vi "Furnace PID Furnance only 20150313.vi"(6 "PID gains":T1={"proportional gain (Kc)"=1.0, "integral time (Ti, min)"=0.1, "derivative time (Td, min)"=0.0}, 9 "PV Furnace degC":dbl format="%.2f", 11 "SP Furnace DegC":dbl format="%.2f") -> (2 "Furnace SP":dbl format="%.2f")   [LabVIEW 2014]
uses:
  <vilib>/addons/control/pid/pid.llb/PID (DBL).vi
  <vilib>/addons/control/pid/NI_PID_pid.lvlib
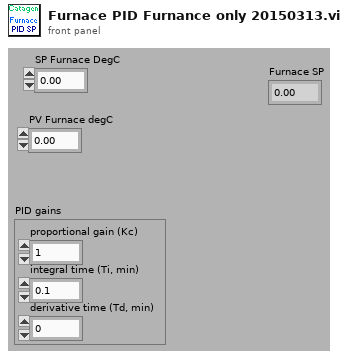
[diagram p1: front panel]
types:
  T1 = cluster{"proportional gain (Kc)":dbl, "integral time (Ti, min)":dbl, "derivative time (Td, min)":dbl}
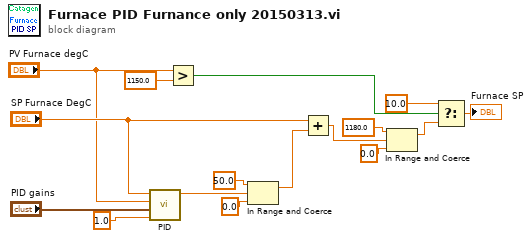
[diagram p0: block diagram]
diagram:
  n1 = call-poly <vilib>:"PID.vi"("dt (s)"=1.0, "PID gains"="PID gains", "process variable"="PV Furnace degC", "setpoint"="SP Furnace DegC") -> ("output"=w8:dbl)  [unwired: 6 in, 1 out]
  n2 = Greater?(x="PV Furnace degC", y=1150.0) -> (0:w10:bool)
  n3 = In Range and Coerce(upper limit=50.0, x=w8, lower limit=0.0) -> (coerced(x)=w7:dbl)  [unwired: 1 out]
  n4 = Add(x="SP Furnace DegC", y=w7) -> (x+y=w3:dbl)
  n5 = In Range and Coerce(upper limit=1180.0, x=w3, lower limit=0.0) -> (coerced(x)=w2:dbl)  [unwired: 1 out]
  n6 = Select(t=10.0, s=w10, f=w2) -> (s? t:f=→"Furnace SP":dbl)
